vi "RT Loop - Acquisition and Logging V1 Config.vi"(8 "error in (no error)":errorcluster, 9 "Acquisition and Logging Configuration":T1={"Data Rate"=1, "Samples per Read"=0, "Number of Reads to Save"=0, "Data File Name"="", "TDMS Properties"=[], "Number of Channels"=4, "Channel Scale Array"=[0.0, 0.0, 0.0, 0.0, 1.0, 1.0, 1.0, 1.0, 1.0, 1.0, 1.0, 1.0, 1.0, 1.0, 1.0, 1.0, 1.0, 1.0, 1.0, 1.0, 1.0, 1.0, 1.0, 1.0], "Channel Names"=[], "Trigger - RMS Value"=0.0, "Trigger - Channel"=0, "Trigger - Time (Minute)"=0} {"Data Rate" items=["51.200 kS/s (NI 9234)"=1, "25.600 kS/s (NI 9234)"=2, "17.067 kS/s (NI 9234)"=3, "12.800 kS/s (NI 9234)"=4, "10.240 kS/s (NI 9234)"=5, "8.533 kS/s (NI 9234)"=6, "7.314 kS/s (NI 9234)"=7, "6.400 kS/s (NI 9234)"=8, "5.689 kS/s (NI 9234)"=9, "5.120 kS/s (NI 9234)"=10, "4.654 kS/s (NI 9234)"=11, "4.267 kS/s (NI 9234)"=12, "3.938 kS/s (NI 9234)"=13, "3.657 kS/s (NI 9234)"=14, "3.413 kS/s (NI 9234)"=15, "3.200 kS/s (NI 9234)"=16, "3.012 kS/s (NI 9234)"=17, "2.845 kS/s (NI 9234)"=18, "2.695 kS/s (NI 9234)"=19, "2.560 kS/s (NI 9234)"=20, "2.438 kS/s (NI 9234)"=21, "2.328 kS/s (NI 9234)"=22, "2.226 kS/s (NI 9234)"=23, "2.133 kS/s (NI 9234)"=24, "2.048 kS/s (NI 9234)"=25, "1.969 kS/s (NI 9234)"=26, "1.896 kS/s (NI 9234)"=27, "1.829 kS/s (NI 9234)"=28, "1.765 kS/s (NI 9234)"=29, "1.707 kS/s (NI 9234)"=30, "1.652 kS/s (NI 9234)"=31]}, 10 "Acquisition and Logging Queue":refnum<queue>, 11 "Message Queue":refnum<queue>) -> ()   [LabVIEW 2015]
uses:
  support/Message Queue/Message Cluster.ctl
  controls/Acquisition and Logging Configuration.ctl
  <vilib>/LabVIEW Targets/FPGA/cRIO/shared/nicrio_ModuleControls/nicrio_cRIO-9234_DataRatesRing2.ctl
  controls/TDMS Properties.ctl
  controls/FPGA VI Reference.ctl
  Globals/Global - Configuration Options.vi
  Globals/Global - Monitoring Variables.vi
  support/Message Queue/Message Queue.lvlib
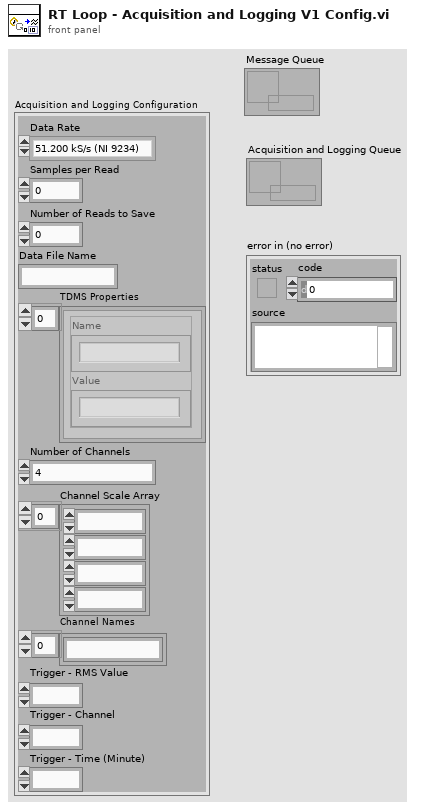
[diagram p1: front panel]
types:
  T1 = typedef "Acquisition and Logging Configuration.ctl" = cluster{"Data Rate":T2, "Samples per Read":i32, "Number of Reads to Save":i32, "Data File Name":string, "TDMS Properties":T3[], "Number of Channels":i32, "Channel Scale Array":fxp<+,24,12>[], "Channel Names":string[], "Trigger - RMS Value":dbl, "Trigger - Channel":i32, "Trigger - Time (Minute)":i32}
  T2 = typedef "nicrio_cRIO-9234_DataRatesRing2.ctl" = u8
  T3 = typedef "TDMS Properties.ctl" = cluster{"Name":string, "Value":string}
  T4 = typedef "FPGA VI Reference.ctl" = refnum<k20>
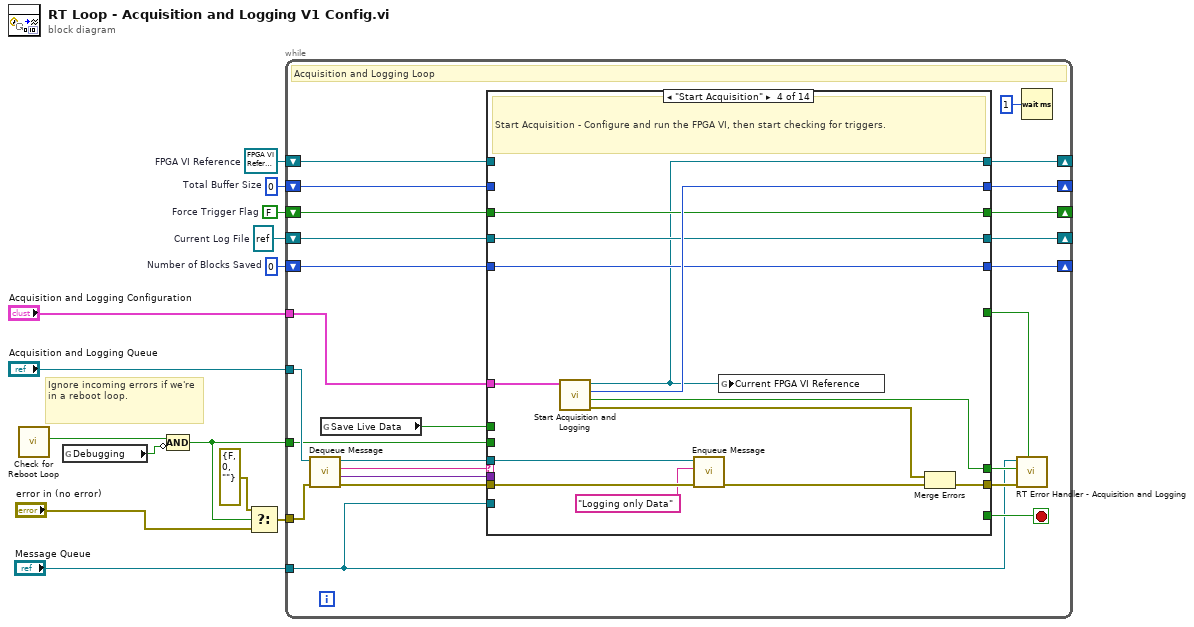
[diagram p0: block diagram]
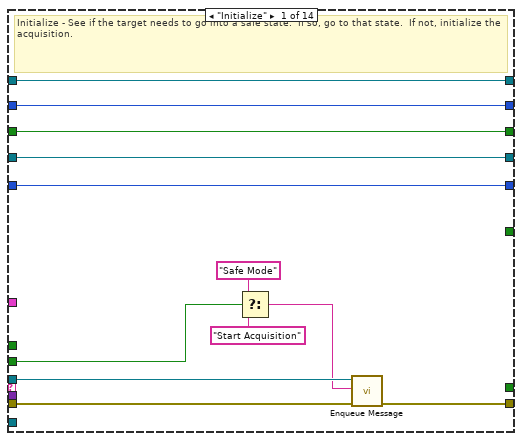
[diagram p2: hidden frame]
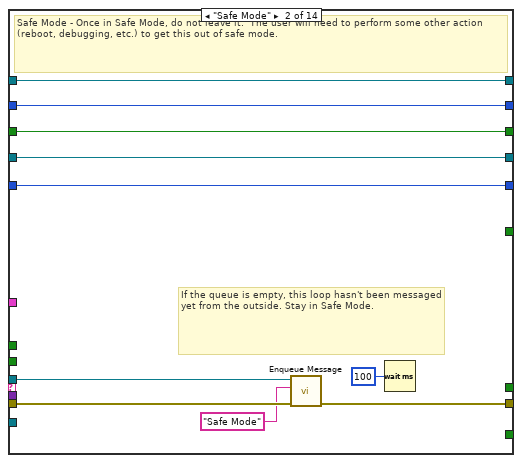
[diagram p3: hidden frame]
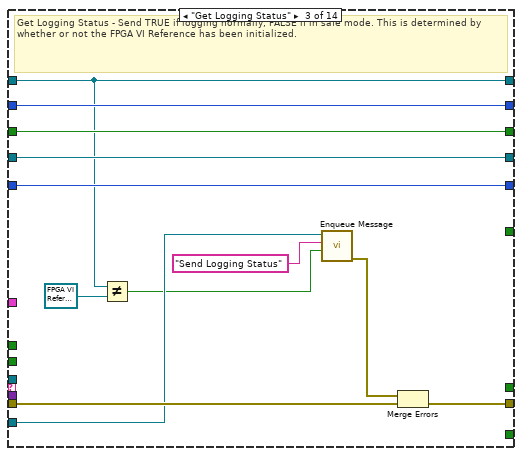
[diagram p4: hidden frame]
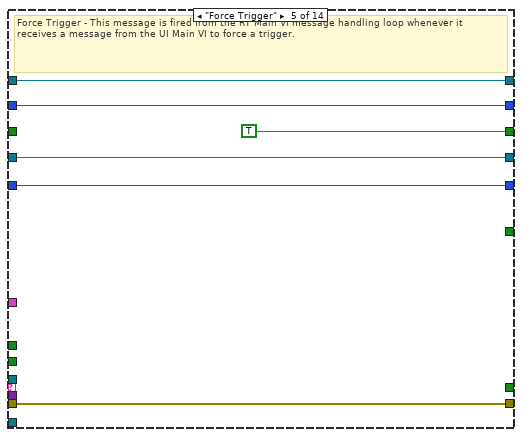
[diagram p5: hidden frame]
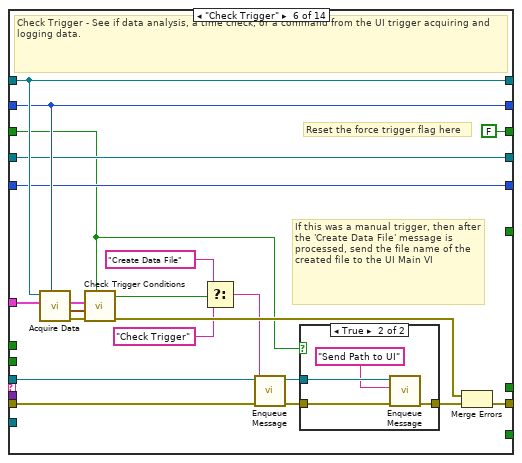
[diagram p6: hidden frame]
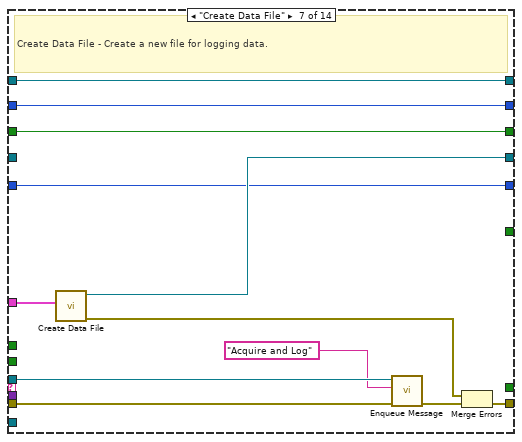
[diagram p8: hidden frame]
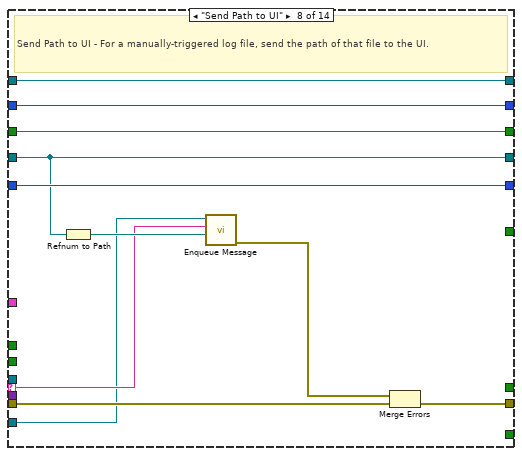
[diagram p9: hidden frame]
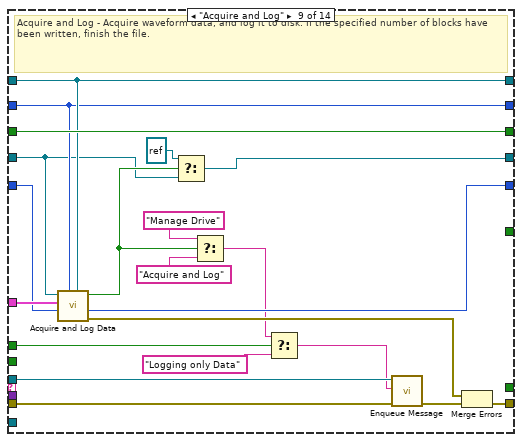
[diagram p10: hidden frame]
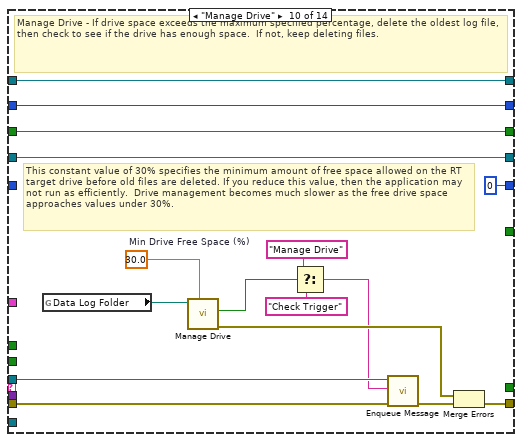
[diagram p11: hidden frame]
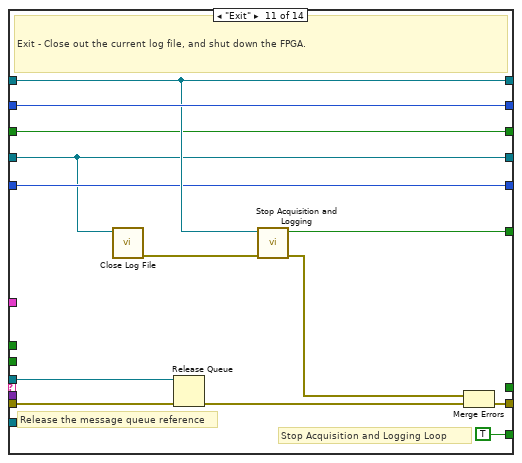
[diagram p12: hidden frame]
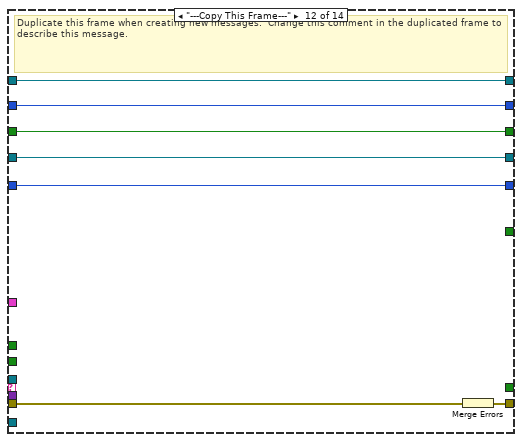
[diagram p13: hidden frame]
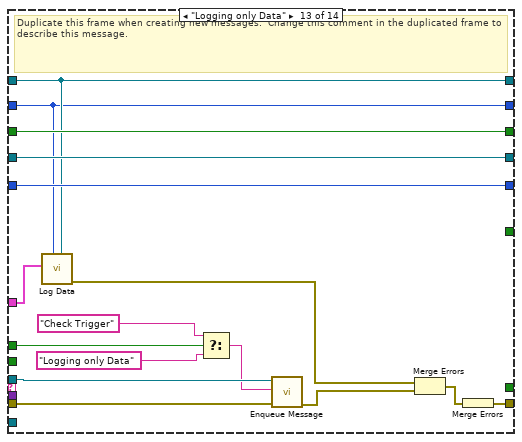
[diagram p14: hidden frame]
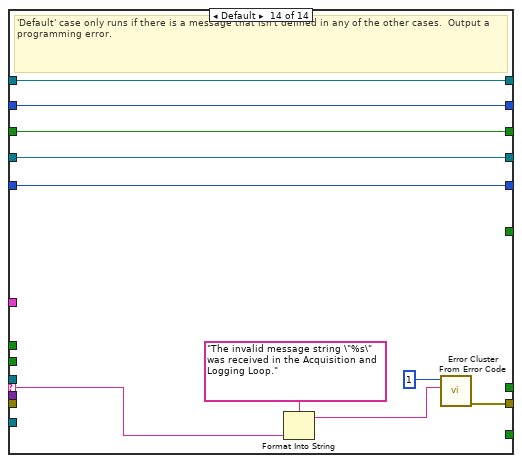
[diagram p15: hidden frame]
diagram:
  w7 = 0  # Number of Blocks Saved
  w8 = refnum<k34> refnum  # Current Log File
  w9 = FALSE  # Force Trigger Flag
  w11 = 0  # Total Buffer Size
  w12 = T4 refnum  # FPGA VI Reference
  # "Ignore incoming errors if we're in a reboot loop."
  n1 = call "Check for Reboot Loop.vi"() -> ("Start in Safe Mode?"=w3:bool)  [unwired: 10 in, 1 out]
  n2 = global read "Global - Configuration Options.vi" "Debugging"() -> (w2:bool)
  n3 = Compound Arithmetic op=AND(w3, invert w2) -> (w1:bool)
  n4 = Select(t=errorcluster {"status"=FALSE, "code"=0, "source"=""}, s=w1, f="error in (no error)") -> (s? t:f=w5:errorcluster)
  n5 = while {
    tunnel: "Acquisition and Logging Queue" -> [w35]
    tunnel: "Message Queue" -> [w19]
    shift-right: [w30] -> _
    shift-left: w12 -> [w32]
    shift-right: [w29] -> _
    shift-left: w11 -> [w31]
    tunnel: "Acquisition and Logging Configuration" -> [w28]
    shift-right: [w24] -> _
    shift-left: w9 -> [w25]
    shift-right: [w22] -> _
    shift-left: w8 -> [w23]
    shift-right: [w20] -> _
    shift-left: w7 -> [w21]
    tunnel: w5 -> [w17]
    tunnel: w1 -> [w16]
    stop <- w39 stop-if-true
    # "Acquisition and Logging Loop"
    n6 = call "Dequeue Message.vi"("error in (no error)"=w17, "Message Queue"=w35) -> ("error out"=w38:errorcluster, "Message Data"=w36:variant, "Message"=w37:string, "dup Message Queue"=w33:refnum<queue>)  [unwired: 6 in]
    n7 = global read "Global - Monitoring Variables.vi" "Save Live Data"() -> (w15:bool)
    n8 = case "Message Cases" shown="\"Start Acquisition\"" w37 {
      selector: w37 -> [_ _ _ _ _ _ _ w134 _ _ _ _ _ w223]
      tunnel: w33 -> [w48 w58 _ w79 _ w104 w125 _ w159 w171 w191 _ w210 _]
      tunnel: w38 -> [w49 w59 w73 w86 w92 w112 w129 w141 w162 w178 w187 w198 w207 _]
      tunnel: [w41 w57 w65 w84 w92 w111 w128 w132 w161 w174 w188 w197 w214 w221] -> w34
      tunnel: [_ _ _ _ _ _ _ _ _ _ TRUE _ _ _] -> w39
      tunnel: w36 -> [_ _ _ _ _ _ _ _ _ _ _ _ _ _]
      tunnel: w32 -> [w51 w61 w68 _ w91 w113 w130 w140 w153 w177 w185 w196 w205 w219]
      tunnel: w31 -> [w50 w60 w72 _ w90 w109 w127 w139 w152 w176 w186 w195 w203 w218]
      tunnel: [w51 w61 w68 w74 w91 w113 w130 w140 w153 w177 w185 w196 w205 w219] -> w30
      tunnel: [w50 w60 w72 w81 w90 w109 w127 w139 w152 w176 w186 w195 w203 w218] -> w29
      tunnel: w28 -> [_ _ _ w85 _ w110 w122 _ w157 _ _ _ w204 _]
      tunnel: [_ _ _ w82 _ _ _ _ _ _ _ _ _ _] -> w26
      tunnel: w25 -> [w44 w56 w71 w77 _ w93 w123 w138 w158 w164 w183 w194 w213 w217]
      tunnel: [w44 w56 w71 w77 TRUE ("Force Trigger Flag") FALSE ("Force Trigger Flag") w123 w138 w158 w164 w183 w194 w213 w217] -> w24
      tunnel: w23 -> [w43 w55 w70 w76 w89 w99 _ w136 w148 w175 w180 w193 w212 w216]
      tunnel: [w43 w55 w70 w76 w89 w99 w120 w136 w147 w175 w180 w193 w212 w216] -> w22
      tunnel: w21 -> [w42 w54 w69 w75 w87 w98 w119 w137 w151 _ w182 w192 w211 w215]
      tunnel: [w42 w54 w69 w75 w87 w98 w119 w137 w150 0 ("Number of Blocks Saved") w182 w192 w211 w215] -> w20
      tunnel: w19 -> [_ _ w66 _ _ _ _ w133 _ _ _ _ _ _]
      tunnel: [_ _ _ _ _ _ _ _ _ _ w179 _ _ _] -> w18
      tunnel: w16 -> [w40 _ _ _ _ _ _ _ _ _ _ _ _ _]
      tunnel: w15 -> [_ _ _ _ _ _ _ _ w145 _ _ _ w200 _]
      frame "Initialize" {
        # "Initialize - See if the target needs to go into a safe state.  If so, go to that state.  If not, initialize the acquisition."
        n9 = Select(t="Safe Mode", s=w40, f="Start Acquisition") -> (s? t:f=w45:string)
        n10 = call "Enqueue Message.vi"("error in (no error)"=w49, "Message"=w45, "Message Queue"=w48) -> ("error out"=w41:errorcluster)  [unwired: 7 in, 1 out]
      }
      frame "Safe Mode" {
        # "If the queue is empty, this loop hasn't been messaged yet from the outside. Stay in Safe Mode."
        # "Safe Mode - Once in Safe Mode, do not leave it.  The user will need to perform some other action (reboot, debugging, etc.) to get this out of safe mode."
        n11 = call "Enqueue Message.vi"("error in (no error)"=w59, "Message"="Safe Mode", "Message Queue"=w58) -> ("error out"=w57:errorcluster)  [unwired: 7 in, 1 out]
        n12 = Wait (ms)(milliseconds to wait=u32 100) -> ()  [unwired: 1 out]
      }
      frame "Get Logging Status" {
        # "Get Logging Status - Send TRUE if logging normally, FALSE if in safe mode. This is determined by whether or not the FPGA VI Reference has been initialized."
        n13 = Not Equal?(x=w68, y=T4 refnum ("FPGA VI Reference")) -> (x != y?=w63:bool)
        n14 = call "Enqueue Message.vi"("Message Data"=w63, "Message"="Send Logging Status", "Message Queue"=w66) -> ("error out"=w64:errorcluster)  [unwired: 7 in, 1 out]
        n15 = Merge Errors(w64, w73) -> (w65:errorcluster)
      }
      frame "Start Acquisition" {
        # "Start Acquisition - Configure and run the FPGA VI, then start checking for triggers."
        n16 = call "Start Acquisition and Logging.vi"("Acquisition and Logging Configuration"=w85) -> ("error out"=w83:errorcluster, "Wait on IRQ Timeout?"=w82:bool, "Total Buffer Size"=w81:i32, "FPGA VI Reference Out"=w74:T4)  [unwired: 7 in]
        n17 = call "Enqueue Message.vi"("error in (no error)"=w86, "Message"="Logging only Data", "Message Queue"=w79) -> ("error out"=w80:errorcluster)  [unwired: 7 in, 1 out]
        n18 = global write "Global - Monitoring Variables.vi" "Current FPGA VI Reference"(w74) -> ()
        n19 = Merge Errors(w83, w80) -> (w84:errorcluster)
      }
      frame "Force Trigger" {
        # "Force Trigger - This message is fired from the RT Main VI message handling loop whenever it receives a message from the UI Main VI to force a trigger."
      }
      frame "Check Trigger" {
        # "If this was a manual trigger, then after the 'Create Data File' message is processed, send the file name of the created file to the UI Main VI"
        # "Reset the force trigger flag here"
        # "Check Trigger - See if data analysis, a time check, or a command from the UI trigger acquiring and logging data."
        n20 = call "Acquire Data.vi"("Total Buffer Size"=w109, "Acquisition and Logging Configuration"=w110, "FPGA VI Reference"=w113) -> ("error out"=w107:errorcluster, "Waveform Data"=w106:waveform(sgl)[], "dup Acquisition and Logging Configuration"=w105:T1)  [unwired: 6 in]
        n21 = call "Check Trigger Conditions.vi"("Force Trigger?"=w93, "error in (no error)"=w107, "Waveform Data"=w106, "Acquisition and Logging Configuration"=w105) -> ("error out"=w108:errorcluster, "Trigger Condition Met?"=w103:bool)  [unwired: 6 in]
        n22 = Select(t="Create Data File", s=w103, f="Check Trigger") -> (s? t:f=w100:string)
        n23 = call "Enqueue Message.vi"("error in (no error)"=w112, "Message"=w100, "Message Queue"=w104) -> ("error out"=w96:errorcluster, "dup Message Queue"=w94:refnum<queue>)  [unwired: 7 in]
        n24 = case shown="True" w93 {
          tunnel: w96 -> [w114 w117]
          tunnel: [w114 w118] -> w95
          tunnel: w94 -> [_ w116]
          frame False {
          }
          frame True {
            n25 = call "Enqueue Message.vi"("error in (no error)"=w117, "Message"="Send Path to UI", "Message Queue"=w116) -> ("error out"=w118:errorcluster)  [unwired: 7 in, 1 out]
          }
        }
        n26 = Merge Errors(w108, w95) -> (w111:errorcluster)
      }
      frame "Create Data File" {
        # "Create Data File - Create a new file for logging data."
        n27 = call "Create Data File.vi"("Acquisition and Logging Configuration"=w122) -> ("error out"=w121:errorcluster, "TDMS File Reference"=w120:refnum<k34>)  [unwired: 9 in]
        n28 = call "Enqueue Message.vi"("error in (no error)"=w129, "Message"="Acquire and Log", "Message Queue"=w125) -> ("error out"=w126:errorcluster)  [unwired: 7 in, 1 out]
        n29 = Merge Errors(w121, w126) -> (w128:errorcluster)
      }
      frame "Send Path to UI" {
        # "Send Path to UI - For a manually-triggered log file, send the path of that file to the UI."
        n30 = Refnum to Path(1:w136) -> (0:w135:path)
        n31 = call "Enqueue Message.vi"("Message Data"=w135, "Message"=w134, "Message Queue"=w133) -> ("error out"=w131:errorcluster)  [unwired: 7 in, 1 out]
        n32 = Merge Errors(w131, w141) -> (w132:errorcluster)
      }
      frame "Acquire and Log" {
        # "Acquire and Log - Acquire waveform data, and log it to disk. If the specified number of blocks have been written, finish the file."
        n33 = call "Acquire and Log Data.vi"("FPGA VI Reference"=w153, "Total Buffer Size"=w152, "Number of Blocks Saved in"=w151, "Acquisition and Logging Configuration"=w157, "TDMS File Reference"=w148) -> ("error out"=w156:errorcluster, "Number of Blocks Saved out"=w150:i32, "Logging Complete?"=w149:bool)  [unwired: 4 in]
        n34 = Select(t=refnum<k34> refnum, s=w149, f=w148) -> (s? t:f=w147:refnum<k34>)
        n35 = Select(t="Manage Drive", s=w149, f="Acquire and Log") -> (s? t:f=w143:string)
        n36 = Select(t=w143, s=w145, f="Logging only Data") -> (s? t:f=w142:string)
        n37 = call "Enqueue Message.vi"("error in (no error)"=w162, "Message"=w142, "Message Queue"=w159) -> ("error out"=w160:errorcluster)  [unwired: 7 in, 1 out]
        n38 = Merge Errors(w156, w160) -> (w161:errorcluster)
      }
      frame "Manage Drive" {
        w173 = 30.0  # Min Drive Free Space (%)
        # "This constant value of 30% specifies the minimum amount of free space allowed on the RT target drive before old files are deleted. If you reduce this value, then the application may not run as efficiently.  Drive management becomes much slower as the free drive space approaches values under 30%."
        # "Manage Drive - If drive space exceeds the maximum specified percentage, delete the oldest log file, then check to see if the drive has enough space.  If not, keep deleting files."
        n39 = global read "Global - Configuration Options.vi" "Data Log Folder"() -> (w163:path)
        n40 = call "Manage Drive.vi"("Min Drive Free Space (%)"=w173, "Data Folder"=w163) -> ("error out"=w170:errorcluster, "Drive Space Below Limit"=w169:bool)  [unwired: 8 in]
        n41 = Select(t="Manage Drive", s=w169, f="Check Trigger") -> (s? t:f=w166:string)
        n42 = call "Enqueue Message.vi"("error in (no error)"=w178, "Message"=w166, "Message Queue"=w171) -> ("error out"=w172:errorcluster)  [unwired: 7 in, 1 out]
        n43 = Merge Errors(w170, w172) -> (w174:errorcluster)
      }
      frame "Exit" {
        # "Stop Acquisition and Logging Loop"
        # "Release the message queue reference"
        # "Exit - Close out the current log file, and shut down the FPGA."
        n44 = call "Close Log File.vi"("Log File"=w180) -> ("error out"=w181:errorcluster)  [unwired: 10 in]
        n45 = Release Queue(queue=w191, error in (no error)=w187) -> (error out=w189:errorcluster)  [unwired: 1 in, 2 out]
        n46 = call "Stop Acquisition and Logging.vi"("error in (no error)"=w181, "FPGA VI Reference"=w185) -> ("error out"=w184:errorcluster, "Stop FPGA Timeout?"=w179:bool)  [unwired: 8 in]
        n47 = Merge Errors(w184, w189) -> (w188:errorcluster)
      }
      frame "---Copy This Frame---" {
        # "Duplicate this frame when creating new messages.  Change this comment in the duplicated frame to describe this message."
        n48 = Merge Errors(w198) -> (w197:errorcluster)
      }
      frame "Logging only Data" {
        # "Duplicate this frame when creating new messages.  Change this comment in the duplicated frame to describe this message."
        n49 = call "Log Data.vi"("FPGA VI Reference"=w205, "Total Buffer Size"=w203, "Acquisition and Logging Configuration"=w204) -> ("error out"=w206:errorcluster)  [unwired: 8 in]
        n50 = Select(t="Check Trigger" ("Message"), s=w200, f="Logging only Data" ("Message")) -> (s? t:f=w201:string)
        n51 = call "Enqueue Message.vi"("error in (no error)"=w207, "Message"=w201, "Message Queue"=w210) -> ("error out"=w209:errorcluster)  [unwired: 7 in, 1 out]
        n52 = Merge Errors(w206, w209) -> (w208:errorcluster)
        n53 = Merge Errors(w208) -> (w214:errorcluster)
      }
      frame Default {
        # "'Default' case only runs if there is a message that isn't defined in any of the other cases.  Output a programming error."
        n54 = Format Into String(format string="The invalid message string \"%s\" was received in the Acquisition and Logging Loop." ("Unknown Message Error Text"), w223) -> (resulting string=w220:string)  [unwired: 2 in, 1 out]
        n55 = call <vilib>:"Error Cluster From Error Code.vi"("error message (\"\")"=w220, "error code (0)"=1) -> ("error out"=w221:errorcluster)  [unwired: 7 in]
      }
    }
    n56 = call "RT Error Handler - Acquisition and Logging.vi"("Stop FPGA Timeout"=w18, "error in (no error)"=w34, "IRQ Timeout"=w26, "Message Queue"=w19) -> ()  [unwired: 7 in, 1 out]
    n57 = Wait (ms)(milliseconds to wait=u32 1) -> ()  [unwired: 1 out]
  }
